vi "random.vi"() -> ()   [LabVIEW 2020]
panel:
  out "Œrednia niby no ale co ja tam umiem":dbl[][](graph)
  out "Obecnie wylosowany punkt":dbl
  out "Œrednia":dbl
  out "Wylosowane liczby":cluster{i32, dbl}(graph)
  out "Array 2":dbl[](array[numeric])
  out "Waveform Graph 2":i32[](graph)
  out "Œrednia":dbl
  out "Waveform Chart":dbl[][](graph)
  out "min index(es)":i32
  out "max index(es)":i32
  out "Wartoœæ min":dbl
  out "Wartoœæ max":dbl
  out "Co wylosowano?":dbl[](array[numeric])
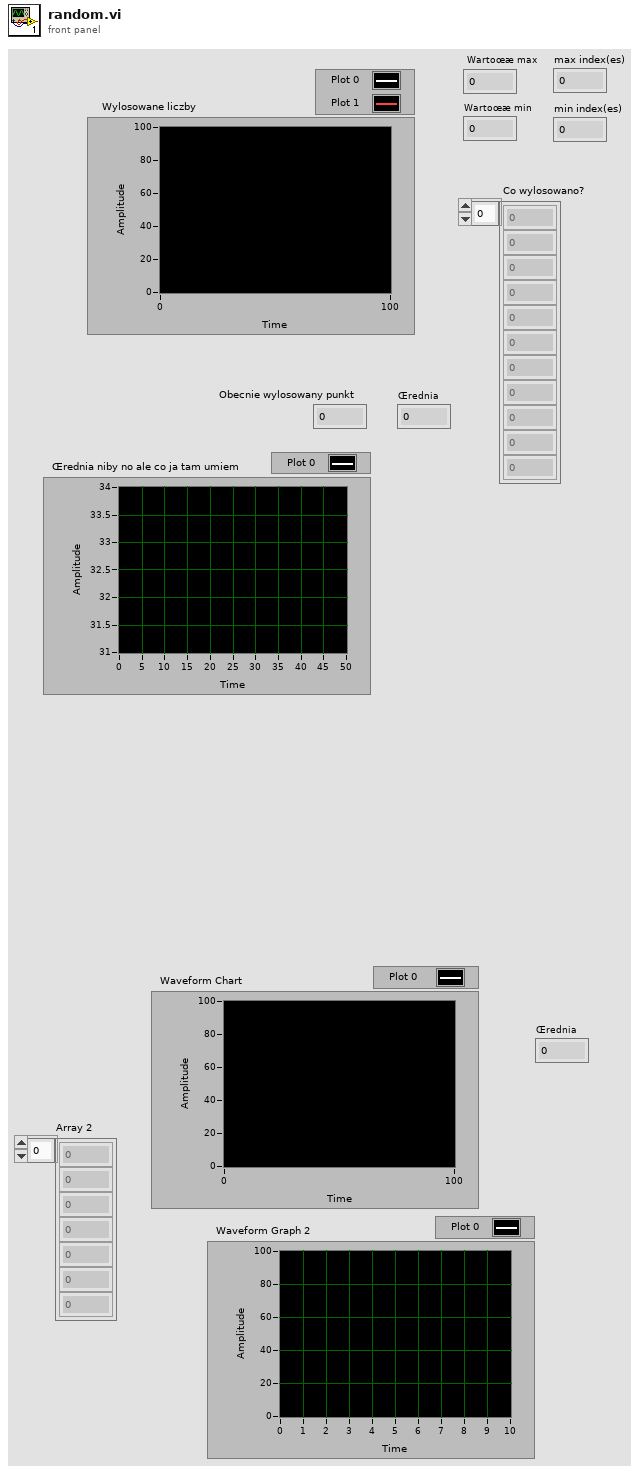
[diagram p1: front panel]
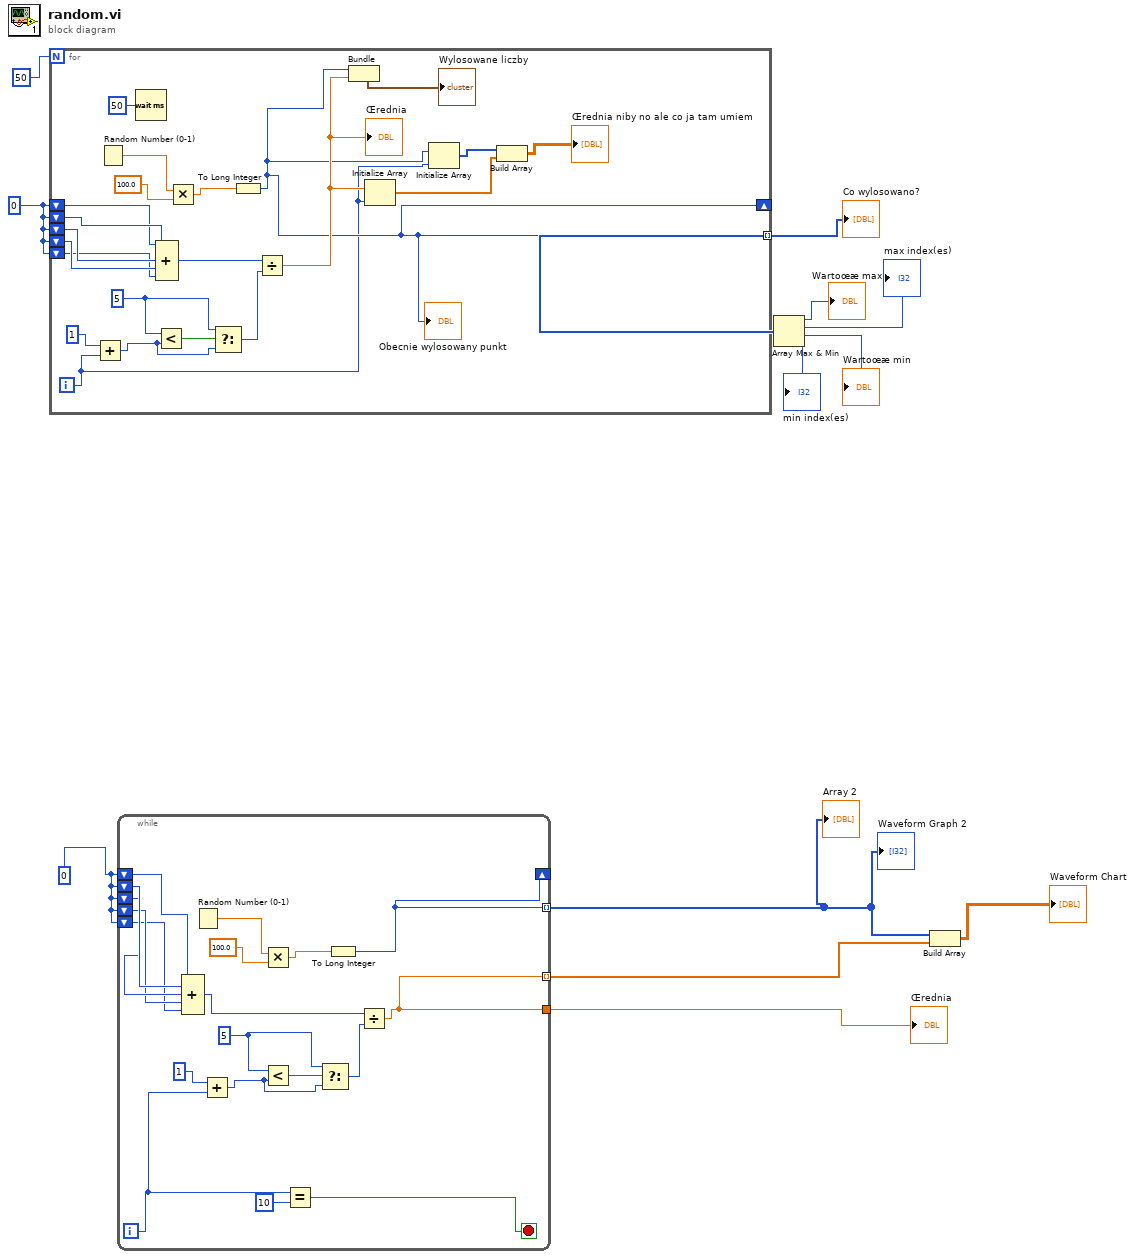
[diagram p0: block diagram]
diagram:
  w7 = 0
  w8 = 0
  n1 = for {
    N: 50 -> [_]
    tunnel: [w17] -> w1 mode=indexing
    shift-right: [w17] -> _
    shift-left: w8 -> [w20]
    shift-left: w8 -> [w30]
    shift-left: w8 -> [w29]
    shift-left: w8 -> [w28]
    shift-left: w8 -> [w27]
    i -> [w16]
    w23 = 5 ("y")
    n2 = Add(x=1, y=w16) -> (x+y=w24:i32)
    n3 = Random Number (0-1)() -> (number: 0 to 1=w33:dbl)
    n4 = Wait (ms)(milliseconds to wait=u32 50) -> ()  [unwired: 1 out]
    n5 = Compound Arithmetic op=ADD(w20, w30, w29, w28, w27) -> (w31:i32)
    n6 = Less?(x=w23, y=w24) -> (x < y?=w25:bool)
    n7 = Multiply(x=w33, y=100.0) -> (x*y=w32:dbl)
    n8 = Select(t=w23, s=w25, f=w24) -> (s? t:f=w22:i32)
    n9 = To Long Integer(number=w32) -> (32bit integer=w17:i32)
    "Obecnie wylosowany punkt" <- w17
    n10 = Divide(x=w31, y=w22) -> (x/y=w18:dbl)
    "Œrednia" <- w18
    n11 = Bundle(w17, w18) -> (→"Wylosowane liczby":cluster{i32, dbl})  [unwired: 1 in]
    n12 = Initialize Array(w18, w16) -> (w14:dbl[])
    n13 = Initialize Array(w17, w16) -> (w15:i32[])
    n14 = Build Array(w15, w14) -> (→"Œrednia niby no ale co ja tam umiem":dbl[][])
  }
  "Co wylosowano?" <- w1
  n15 = while {
    shift-right: [w36] -> _
    shift-left: w7 -> [w43]
    shift-left: w7 -> [w42]
    shift-left: w7 -> [w41]
    shift-left: w7 -> [w40]
    shift-left: w7 -> [w39]
    tunnel: [w35] -> w6
    tunnel: [w36] -> w3 mode=indexing
    tunnel: [w35] -> w5 mode=indexing
    i -> [w44]
    stop <- w49 stop-if-true
    w45 = 5 ("y")
    n16 = Compound Arithmetic op=ADD(w43, w42, w41, w40, w39) -> (w38:i32)
    n17 = Random Number (0-1)() -> (number: 0 to 1=w52:dbl)
    n18 = Add(x=1, y=w44) -> (x+y=w46:i32)
    n19 = Multiply(x=w52, y=100.0) -> (x*y=w51:dbl)
    n20 = Less?(x=w45, y=w46) -> (x < y?=w47:bool)
    n21 = Equal?(x=w44, y=10) -> (x = y?=w49:bool)
    n22 = Select(t=w45, s=w47, f=w46) -> (s? t:f=w37:i32)
    n23 = To Long Integer(number=w51) -> (32bit integer=w36:i32)
    n24 = Divide(x=w38, y=w37) -> (x/y=w35:dbl)
  }
  "Œrednia" <- w6
  "Waveform Graph 2" <- w3
  "Array 2" <- w3
  n25 = Array Max & Min(array=w1) -> (max value=→"Wartoœæ max":i32, max index (indices)=→"max index(es)":i32, min value=→"Wartoœæ min":i32, min index (indices)=→"min index(es)":i32)
  n26 = Build Array(w3, w5) -> (→"Waveform Chart":dbl[][])
